vi "FGV ANA-OUT.vi"(6 "Aktion":T1, 11 "ANA-OUT Gase":sgl[](array[numeric])) -> (3 "ANA-OUT 1-16":sgl[](array[numeric]))   [LabVIEW 2020, in "Gaszuordnung AO.lvlib"]
uses:
  Gaszuordnung AO.lvlib
  ANA-OUT Aktionen.ctl
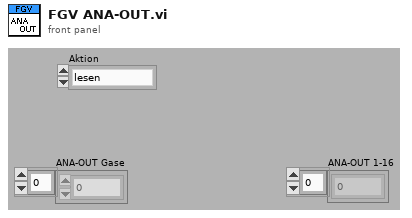
[diagram p1: front panel]
types:
  T1 = typedef "Gaszuordnung AO.lvlib/ANA-OUT Aktionen.ctl" = enum16{"lesen", "Gase schreiben"}
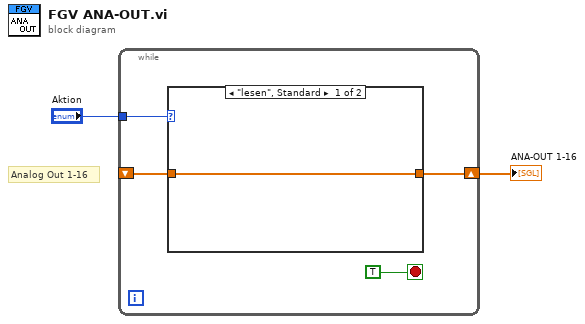
[diagram p0: block diagram]
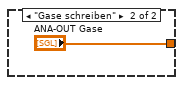
[diagram p2: hidden frame]
diagram:
  # "Analog Out 1-16"
  n1 = while {
    tunnel: "Aktion" -> [w5]
    shift-right: [w4] -> w1
    shift-left: _ -> [w3]
    stop <- TRUE stop-if-true
    n2 = case shown="\"lesen\", Standard" w5 {
      tunnel: [w7 "ANA-OUT Gase"] -> w4
      tunnel: w3 -> [w7 _]
      frame "lesen", Default {
      }
      frame "Gase schreiben" {
      }
    }
  }
  "ANA-OUT 1-16" <- w1
